vi "aal_Error Priority.vi"() -> ()   [LabVIEW 2014, in "NI_AALPro.lvlib"]
uses:
  NI_AALPro.lvlib
panel:
  out "error code":i32
  in  "error codes":i32[](array[numeric])
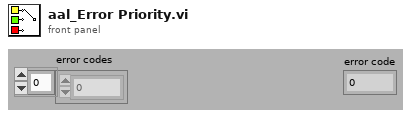
[diagram p1: front panel]
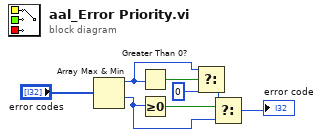
[diagram p0: block diagram]
diagram:
  n1 = Array Max & Min(array="error codes") -> (max value=w4:i32, min value=w6:i32)  [unwired: 2 out]
  n2 = Greater Than 0?(x=w4) -> (x > 0?=w5:bool)
  n3 = Greater Or Equal To 0?(x=w6) -> (x >= 0?=w7:bool)
  n4 = Select(t=w4, s=w5, f=0) -> (s? t:f=w2:i32)
  n5 = Select(t=w2, s=w7, f=w6) -> (s? t:f=→"error code":i32)
